vi "Initialize.vi"(8 "error in (no error)":errorcluster, 9 "Requestor":string, 10 "Requestee":string, 11 "Mag Lab Hardware in":refnum<class "Linear Research.lvclass">) -> (0 "error out":errorcluster, 3 "Mag Lab Hardware out":refnum<class "Linear Research.lvclass">)   [LabVIEW 2015, in "Linear Research.lvclass"]
uses:
  Linear Research.lvclass
  Linear Research.lvclass/Linear Research.ctl
  Meter/Meter.lvclass
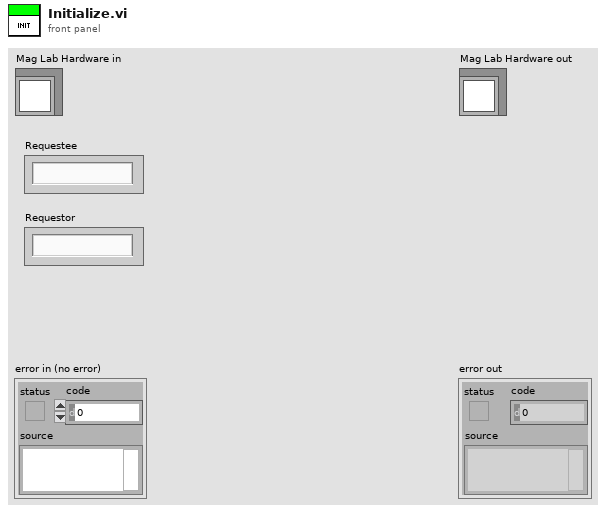
[diagram p1: front panel]
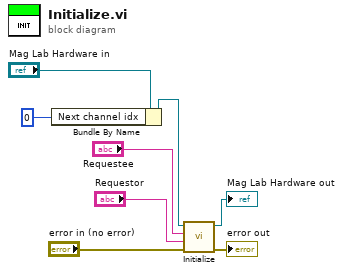
[diagram p0: block diagram]
diagram:
  n1 = Bundle By Name(cluster="Mag Lab Hardware in", "Next channel idx"=0) -> (w2:refnum<class "Linear Research.lvclass">)
  n2 = call-parent "Initialize.vi"("error in (no error)"="error in (no error)", "Requestor"="Requestor", "Requestee"="Requestee", "Mag Lab Hardware in"=w2) -> ("error out"=→"error out":errorcluster, "Mag Lab Hardware out"=→"Mag Lab Hardware out":refnum<class "Linear Research.lvclass">)  [unwired: 6 in]
